vi "Test Copy Image ARGB Mask ARGB.vi"(8 "error in (no error)":errorcluster, 11 "Test Case In":refnum<class "01_Image.lvclass">) -> (0 "error out":errorcluster, 3 "Test Case Out":refnum<class "01_Image.lvclass">)   [LabVIEW 2020, in "test.lvlib" / "01_Image.lvclass"]
uses:
  01_Image.lvclass
  C:/Program Files (x86)/National Instruments/LabVIEW 2026/vi.lib/Astemes/LUnit/Test Case.lvclass
  common/Image Size (Integer).ctl
  <vilib>/Astemes/LUnit/Test Case.lvclass/Test Case.ctl
  image/New Image (ARGB Preallocated).vi
  image/Copy Array to Image (ARGB).vi
  image/Copy Image (ARGB with ARGB Mask).vi
  4993e8ee-a06a-463a-9684-69129f64d5ce.vi
  image/New Image (ARGB Preallocated).vi/3321fa97-f432-4e1e-8db9-a0df79aed21b.vi
  image/ARGB Colour to U32 Pixel Value.vi
  image/Copy Image (ARGB with ARGB Mask).vi/3b1fb24f-4521-4d3d-a8b9-ed3d08148c99.vi
  <vilib>/Astemes/LUnit/Core/LUnit Test Case/Private/Append Pass Result.vi
  <vilib>/Astemes/LUnit/Core/LUnit Test Case/Private/Append Fail Result.vi
  4993e8ee-a06a-463a-9684-69129f64d5ce.vi/9c5d11cd-9439-4240-a1ee-d9baace9c924.vi
  <vilib>/Astemes/LUnit/Core/LUnit Test Case/Private/Run In UI.vi
  <vilib>/Utility/error.llb/Clear Errors.vi
  <vilib>/Utility/error.llb/Error Cluster From Error Code.vi
  <vilib>/picture/pixmap.llb/Flatten Pixmap.vi
  image/image.lvlib
  common/common.lvlib
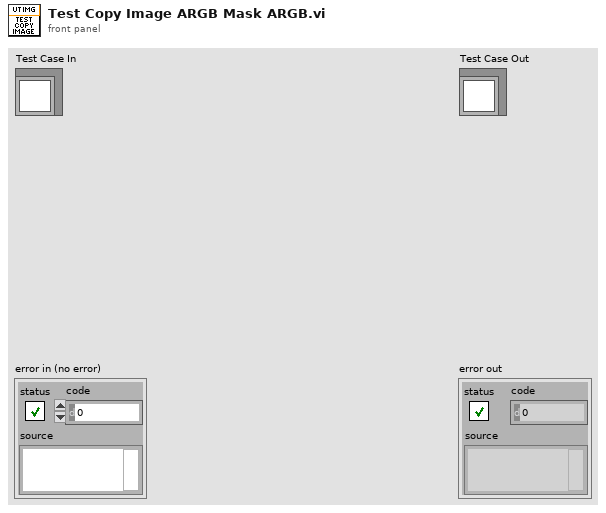
[diagram p1: front panel]
types:
  T1 = typedef "common.lvlib/Image Size (Integer).ctl" = cluster{"Width":u16, "Height":u16}
  T2 = typedef "image.lvlib/ARGB Image.ctl" = refnum<data-value>
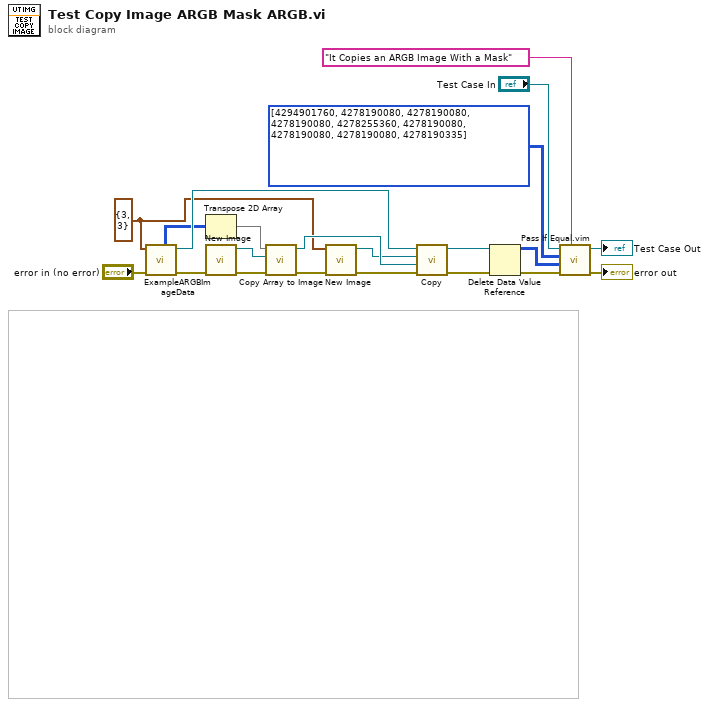
[diagram p0: block diagram]
diagram:
  w3 = T1 {"Width"=3, "Height"=3} ("Preallocated Image Size (Default - 0,0)")
  n1 = call "ExampleARGBImageData.vi"("error in (no error)"="error in (no error)", "Image Size"=w3) -> ("error out"=w16:errorcluster, "Data Value Reference out"=w14:T2, "ARGB Array Data"=w12:u32[][])  [unwired: 6 in, 1 out]
  n2 = Transpose 2D Array(2D array=w12) -> (transposed array=w9:u32[][])
  n3 = call-poly "New Image.vi"("error in (no error)"=w16) -> ("error out"=w11:errorcluster, "ARGB Image"=w8:T2)  [unwired: 9 in]
  n4 = call-poly "Copy Array to Image.vi"("error in (no error)"=w11, "ARGB Image Destination in"=w8, "U32 ARBG Data"=w9) -> ("error out"=w10:errorcluster, "ARGB Image Destination"=w7:T2)  [unwired: 7 in]
  n5 = call-poly "New Image.vi"("error in (no error)"=w10, "Preallocated Image Size (Default: 0,0)"=w3) -> ("error out"=w5:errorcluster, "ARGB Image"=w6:T2)  [unwired: 8 in]
  n6 = call-poly "Copy.vi"("error in (no error)"=w5, "ARGB Image Mask in"=w7, "ARGB Image Destination in"=w6, "ARGB Image Source in"=w14) -> ("error out"=w4:errorcluster, "ARGB Image Destination"=w13:T2)  [unwired: 6 in]
  n7 = Delete Data Value Reference(data value reference=w13, error in=w4) -> (data value=w2:u32[][], error out=w15:errorcluster)
  n8 = call "Pass If Equal.vim"("Description"="It Copies an ARGB Image With a Mask", "error in (no error)"=w15, "Actual"=w2, "Expected"=u32[][] [[4294901760, 4278190080, 4278190080], [4278190080, 4278255360, 4278190080], [4278190080, 4278190080, 4278190335]] ("data value"), "LUnit Test Case In"="Test Case In") -> ("error out"=→"error out":errorcluster, "LUnit Test Case Out"=→"Test Case Out":refnum<class "01_Image.lvclass">)  [unwired: 5 in]
